vi "Calculate and Update Scalar Results.vi"(9 "ADC codes":u32[][](array[numeric]), 10 "measurement results":T1, 11 "Sweep transition settings":T2) -> (2 "measurement results out":T1)   [LabVIEW 2021, in "Full Scale Error_ADC.lvlib"]
uses:
  Full Scale Error_ADC.lvlib
  Controls/Sweep Transition Settings.ctl
  Measurement Results.ctl
  Controls/ADC Data.ctl
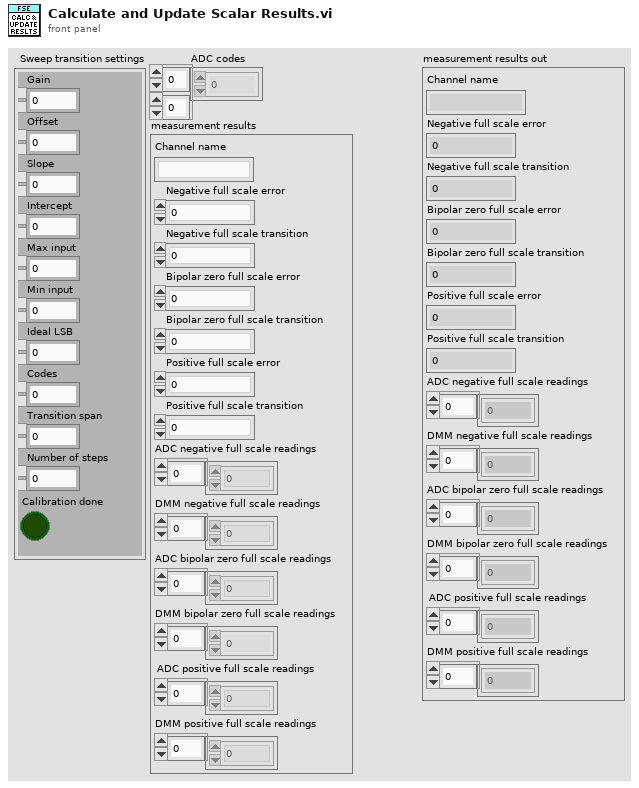
[diagram p1: front panel]
types:
  T1 = typedef "Full Scale Error_ADC.lvlib/Measurement Results.ctl" = cluster{"Channel name":string, "Negative full scale error":dbl, "Negative full scale transition":dbl, "Bipolar zero full scale error":dbl, "Bipolar zero full scale transition":dbl, "Positive full scale error":dbl, "Positive full scale transition":dbl, "ADC negative full scale readings":dbl[], "DMM negative full scale readings":dbl[], "ADC bipolar zero full scale readings":dbl[], "DMM bipolar zero full scale readings":dbl[], "ADC positive full scale readings":dbl[], "DMM positive full scale readings":dbl[]}
  T2 = typedef "Full Scale Error_ADC.lvlib/Sweep Transition Settings.ctl" = cluster{"Gain":dbl, "Offset":dbl, "Slope":dbl, "Intercept":dbl, "Max input":dbl, "Min input":dbl, "Ideal LSB":dbl, "Codes":dbl, "Transition span ":dbl, "Number of steps":i32, "Calibration done":bool}
  T3 = typedef "Full Scale Error_ADC.lvlib/ADC Data.ctl" = cluster{"Measured voltage":dbl, "ADC code":u32, "Scaled ADC code":dbl}
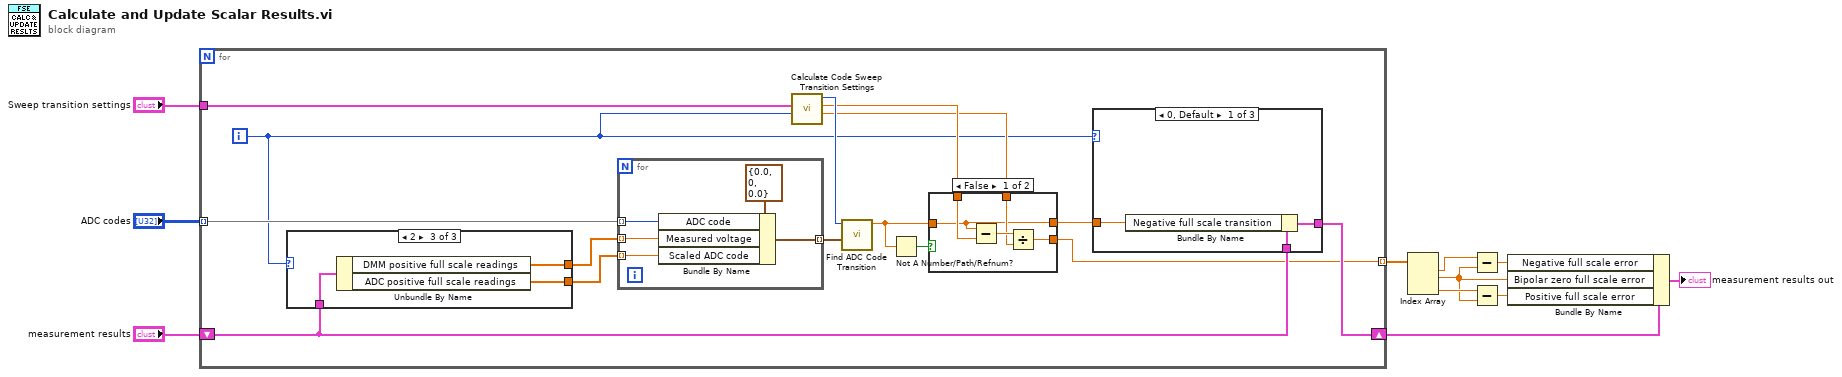
[diagram p0: block diagram]
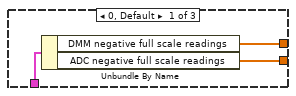
[diagram p2: hidden frame]
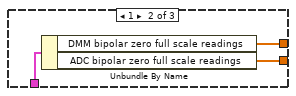
[diagram p3: hidden frame]
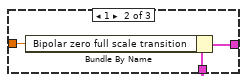
[diagram p4: hidden frame]
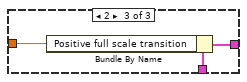
[diagram p5: hidden frame]
diagram:
  n1 = for {
    tunnel: "Sweep transition settings" -> [w22]
    shift-right: [w18] -> w5
    shift-left: "measurement results" -> [w15]
    tunnel: "ADC codes" -> [w17] mode=indexing
    tunnel: [w12] -> w6 mode=indexing
    i -> [w16]
    n2 = case shown="2" w16 {
      tunnel: w15 -> [w29 w32 w35]
      tunnel: [w28 w31 w34] -> w14
      tunnel: [w27 w30 w33] -> w13
      frame 0, Default {
        n3 = Unbundle By Name(w29) -> ("DMM negative full scale readings"=w28:dbl[], "ADC negative full scale readings"=w27:dbl[])
      }
      frame 1 {
        n4 = Unbundle By Name(w32) -> ("DMM bipolar zero full scale readings"=w31:dbl[], "ADC bipolar zero full scale readings"=w30:dbl[])
      }
      frame 2 {
        n5 = Unbundle By Name(w35) -> ("DMM positive full scale readings"=w34:dbl[], "ADC positive full scale readings"=w33:dbl[])
      }
    }
    n6 = for {
      tunnel: w17 -> [w53] mode=indexing
      tunnel: [w54] -> w26 mode=indexing
      tunnel: w14 -> [w52] mode=indexing
      tunnel: w13 -> [w51] mode=indexing
      n7 = Bundle By Name(cluster=T3 {"Measured voltage"=0.0, "ADC code"=0, "Scaled ADC code"=0.0} ("ADC data"), "ADC code"=w53, "Measured voltage"=w52, "Scaled ADC code"=w51) -> (w54:T3)
    }
    n8 = call "Calculate Code Sweep Transition Settings.vi"("Code transition type"=w16, "Sweep transition settings"=w22) -> ("Ideal LSB"=w19:dbl, "Ideal transition"=w20:dbl, "Code before transition"=w21:u32)  [unwired: 6 in, 1 out]
    n9 = call "Find ADC Code Transition.vi"("ADC data"=w26, "code before transition"=w21) -> ("transition voltage"=w24:dbl)  [unwired: 9 in]
    n10 = Not A Number/Path/Refnum?(number/path/refnum=w24) -> (NaN/Path/Refnum?=w23:bool)
    n11 = case shown="False" w23 {
      tunnel: w24 -> [w45 w50]
      tunnel: w20 -> [w46 _]
      tunnel: w19 -> [w48 _]
      tunnel: [w47 w50] -> w12
      tunnel: [w45 w50] -> w25
      frame False {
        n12 = Subtract(x=w45, y=w46) -> (x-y=w49:dbl)
        n13 = Divide(x=w49, y=w48) -> (x/y=w47:dbl)
      }
      frame True {
      }
    }
    n14 = case shown="0, Default" w16 {
      tunnel: w25 -> [w38 w41 w44]
      tunnel: w15 -> [w37 w40 w43]
      tunnel: [w36 w39 w42] -> w18
      frame 0, Default {
        n15 = Bundle By Name(cluster=w37, "Negative full scale transition"=w38) -> (w36:T1)
      }
      frame 1 {
        n16 = Bundle By Name(cluster=w40, "Bipolar zero full scale transition"=w41) -> (w39:T1)
      }
      frame 2 {
        n17 = Bundle By Name(cluster=w43, "Positive full scale transition"=w44) -> (w42:T1)
      }
    }
  }
  n18 = Index Array(array=w6) -> (element #1=w8:dbl, element #2=w2:dbl, element #3=w7:dbl)  [unwired: 3 in]
  n19 = Subtract(x=w8, y=w2) -> (x-y=w3:dbl)
  n20 = Subtract(x=w7, y=w2) -> (x-y=w1:dbl)
  n21 = Bundle By Name(cluster=w5, "Negative full scale error"=w3, "Bipolar zero full scale error"=w2, "Positive full scale error"=w1) -> (→"measurement results out":T1)
